vi "Get condition of date in report.vi"(9 "Date":T1 {"From :" format="%<%d/%m/%y>T"; "To :" format="%<%d/%m/%y>T"}, 10 "Intial condition":string, 11 "Date Label":string) -> (3 "Condition":string)   [LabVIEW 2015]
uses:
  controls/Date to query in report.ctl
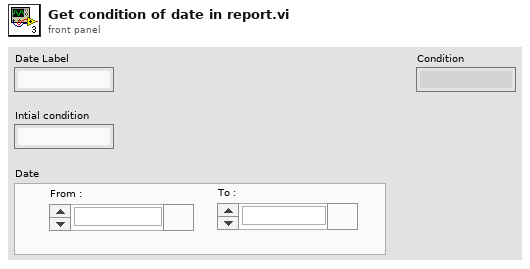
[diagram p1: front panel]
types:
  T1 = typedef "Date to query in report.ctl" = cluster{"To :":timestamp, "From : ":timestamp}
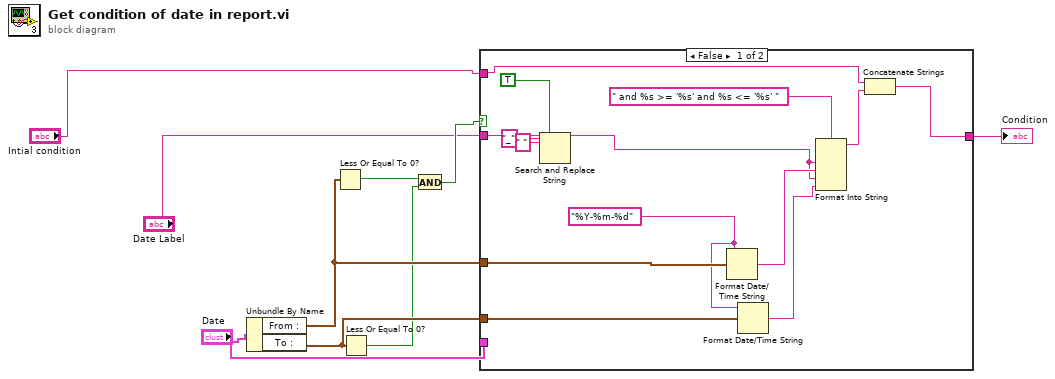
[diagram p0: block diagram]
diagram:
  n1 = Unbundle By Name("Date") -> ("From :"=w8:timestamp, "To :"=w9:timestamp)
  n2 = Less Or Equal To 0?(x=w8) -> (x <= 0?=w6:bool)
  n3 = Less Or Equal To 0?(x=w9) -> (x <= 0?=w5:bool)
  n4 = And(x=w6, y=w5) -> (x .and. y?=w7:bool)
  n5 = case shown="False" w7 {
    tunnel: "Date Label" -> [w22 _]
    tunnel: [w16 w24] -> w2
    tunnel: "Intial condition" -> [w18 w24]
    tunnel: "Date" -> [_ _]
    tunnel: w8 -> [w15 _]
    tunnel: w9 -> [w13 _]
    frame False {
      w14 = "%Y-%m-%d"
      n6 = Search and Replace String(replace all?=TRUE ("replace all? (F)"), input string=w22, search string=" ", replace string="_" ("replace string (\"\")")) -> (result string=w10:string)  [unwired: 4 in, 3 out]
      n7 = Format Date/Time String(time format string (%c)=w14, seconds (now)=w15) -> (date/time string=w11:string)  [unwired: 1 in]
      n8 = Format Date/Time String(time format string (%c)=w14, seconds (now)=w13) -> (date/time string=w12:string)  [unwired: 1 in]
      n9 = Format Into String(format string=" and %s >= '%s' and %s <= '%s' ", w10, w11, w10, w12) -> (resulting string=w17:string)  [unwired: 2 in, 1 out]
      n10 = Concatenate Strings(w18, w17) -> (w16:string)
    }
    frame True {
    }
  }
  "Condition" <- w2
